vi "Send Message.vi"(6 "ID":string, 8 "error in (no error)":errorcluster, 9 "Data":variant, 10 "Command":string, 11 "RemoteControl.ZMQ in":refnum<class "RemoteControl.ZMQ.lvclass">) -> (0 "error out":errorcluster, 3 "RemoteControl.ZMQ out":refnum<class "RemoteControl.ZMQ.lvclass">)   [LabVIEW 2019, in "RemoteControl.ZMQ.lvclass"]
uses:
  RemoteControl.ZMQ.lvclass
  C:/Users/patrick/Documents/GitHub/Instrument-Framework/lvsrc/SMOs/RemoteControl/RemoteControl.lvclass
  RemoteControl.ZMQ.lvclass/RemoteControl.ZMQ.ctl
  RemoteControl/RemoteControl.lvclass/RemoteControl.ctl
  RemoteControl/Typedefs/Message--Cluster.ctl
  RemoteControl/RemoteControl.lvclass
  <userlib>/LevyLab/Instrument Framework/SMOs/JSON-RPC/JSON-RPC/JSON-RPC.lvclass
  <vilib>/addons/zeromq/zmq_socket.lvclass
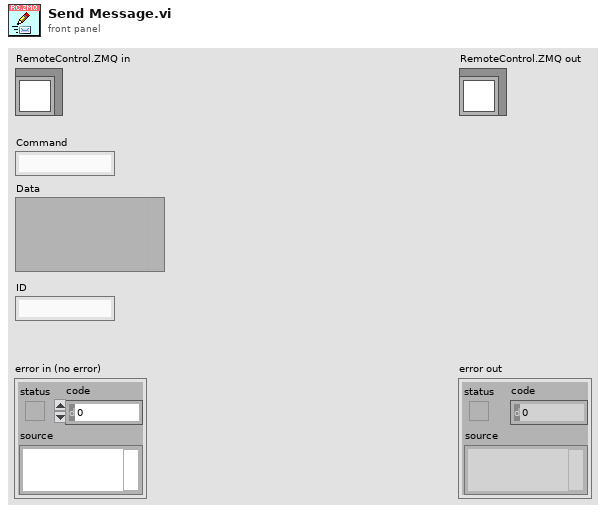
[diagram p1: front panel]
types:
  T1 = typedef "RemoteControl.lvclass/Message--Cluster.ctl" = cluster{"Command":string, "Data":variant, "ID":string}
  T2 = typedef "zeromq.lvlib/socket_type.ctl" = enum8{"ZMQ_PAIR", "ZMQ_PUB", "ZMQ_SUB", "ZMQ_REQ", "ZMQ_REP", "ZMQ_DEALER", "ZMQ_ROUTER", "ZMQ_PULL", "ZMQ_PUSH", "ZMQ_XPUB", "ZMQ_XSUB", "ZMQ_STREAM", "ZMQ_SERVER", "ZMQ_CLIENT", "ZMQ_RADIO", "ZMQ_DISH", "ZMQ_GATHER", "ZMQ_SCATTER", "ZMQ_DGRAM"}
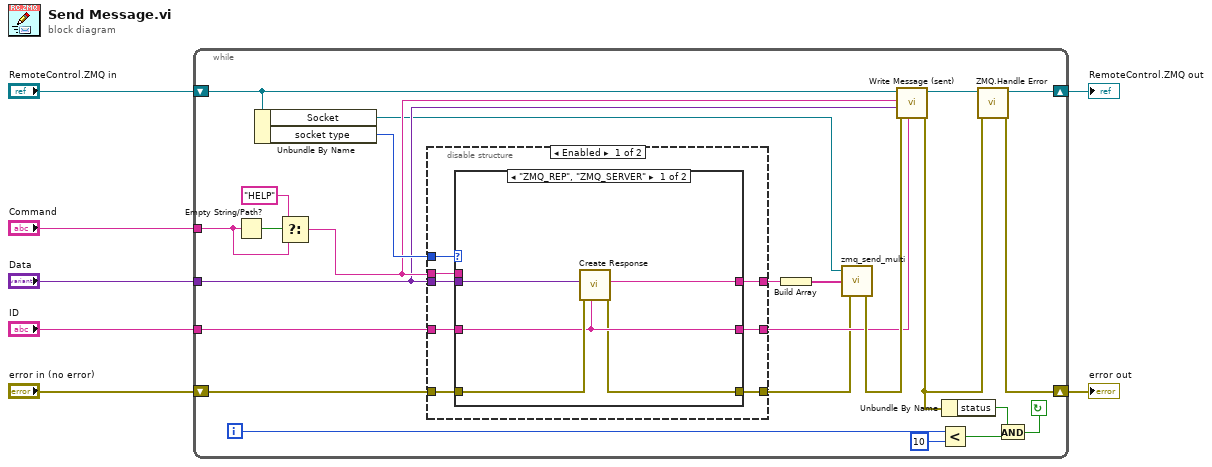
[diagram p0: block diagram]
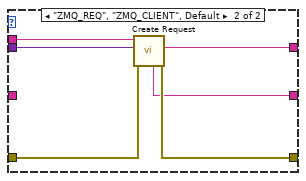
[diagram p2: hidden frame]
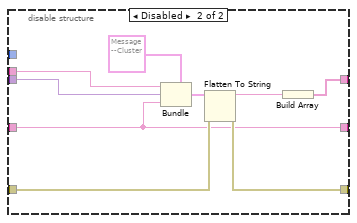
[diagram p3: hidden frame]
diagram:
  n1 = while {
    tunnel: "Command" -> [w14]
    tunnel: "ID" -> [w28]
    tunnel: "Data" -> [w23]
    shift-right: [w16] -> w4
    shift-left: "RemoteControl.ZMQ in" -> [w19]
    shift-right: [w15] -> w3
    shift-left: "error in (no error)" -> [w18]
    i -> [w13]
    stop <- w10 continue-if-true
    n2 = Empty String/Path?(string/path=w14) -> (empty?=w30:bool)
    n3 = Unbundle By Name(w19) -> ("Socket"=w22:refnum<class "zmq_socket.lvclass">, "socket type"=w29:T2)
    n4 = Select(t="HELP", s=w30, f=w14) -> (s? t:f=w27:string)
    n5 = disable-structure shown="Enabled" {
      disable-tunnel: w23 -> [w39 w53]
      disable-tunnel: w27 -> [w38 w54]
      disable-tunnel: [w37 w51] -> w24
      disable-tunnel: w18 -> [w36 w57]
      disable-tunnel: [w35 w56] -> w20
      disable-tunnel: w29 -> [w34 _]
      disable-tunnel: w28 -> [w32 w52]
      disable-tunnel: [w33 w52] -> w25
      frame Enabled {
        n6 = case shown="\"ZMQ_REP\", \"ZMQ_SERVER\"" w34 {
          tunnel: w38 -> [_ w50]
          tunnel: w39 -> [w44 w49]
          tunnel: [w40 w45] -> w37
          tunnel: w36 -> [w43 w48]
          tunnel: [w41 w47] -> w35
          tunnel: w32 -> [w42 _]
          tunnel: [w42 w46] -> w33
          frame "ZMQ_REP", "ZMQ_SERVER" {
            n7 = call <userlib>:"Create Response.vi"("id"=w42, "error in (no error)"=w43, "result"=w44) -> ("error out"=w41:errorcluster, "{JSON} Response"=w40:string)  [unwired: 6 in, 1 out]
          }
          frame "ZMQ_REQ", "ZMQ_CLIENT", Default {
            n8 = call <userlib>:"Create Request.vi"("error in (no error)"=w48, "params"=w49, "method"=w50) -> ("error out"=w47:errorcluster, "{JSON} Requests"=w45:string, "ID"=w46:string)  [unwired: 5 in, 1 out]
          }
        }
      }
      frame Disabled {
        n9 = Bundle(cluster=T1 {"Command"="", "Data"=variant(string ""), "ID"=""} ("Message"), "Command"=w54, "Data"=w53, "ID"=w52) -> (w59:T1)
        n10 = Flatten To String(anything=w59, error in (no error)=w57) -> (data string=w55:string, error out=w56:errorcluster)  [unwired: 2 in, 1 out]
        n11 = Build Array(w55) -> (w51:string[])
      }
    }
    n12 = Build Array(w24) -> (w21:string[])
    n13 = call <vilib>:"zmq_send_multi.vi"("error in"=w20, "parts"=w21, "socket in"=w22) -> ("error out"=w26:errorcluster)  [unwired: 1 in, 1 out]
    n14 = call "Write Message (sent).vi"("ID (sent)"=w25, "error in (no error)"=w26, "Data"=w23, "Command (sent)"=w27, "RemoteControl in"=w19) -> ("error out"=w8:errorcluster, "RemoteControl out"=w17:refnum<class "RemoteControl.ZMQ.lvclass">)  [unwired: 5 in]
    n15 = Less?(x=w13, y=10) -> (x < y?=w11:bool)
    n16 = Unbundle By Name(w8) -> ("status"=w9:bool)
    n17 = call "ZMQ.Handle Error.vi"("error in (no error)"=w8, "RemoteControl.ZMQ in"=w17) -> ("error out"=w15:errorcluster, "RemoteControl.ZMQ out"=w16:refnum<class "RemoteControl.ZMQ.lvclass">)  [unwired: 8 in]
    n18 = And(x=w9, y=w11) -> (x .and. y?=w10:bool)
  }
  "error out" <- w3
  "RemoteControl.ZMQ out" <- w4
